vi "map other module channels.vi"(7 "instance id":string, 9 "channels":refnum<class "TBM channel.lvclass">[](array[class]), 10 "engine configuration in":refnum<class "engine configuration.lvclass">, 11 "TEC configuration in":refnum<class "TEC configuration.lvclass">) -> (0 "error out":errorcluster, 2 "engine configuration out":refnum<class "engine configuration.lvclass">, 3 "TEC configuration out":refnum<class "TEC configuration.lvclass">)   [LabVIEW 2013, in "TEC editor node.lvclass"]
uses:
  TEC editor node.lvclass
  <vilib>/NI/Module Execution Interface/Engine Configuration/engine configuration.lvclass
  configuration/TEC configuration.lvclass
  <vilib>/NI/Tag Bus Module Framework/channel/TBM channel.lvclass
  <vilib>/NI/Tag Bus Module Framework/channel/channel classification.ctl
  <vilib>/NI/Tag Bus Module Framework/channel/TBM channel.lvclass/TBM channel.ctl
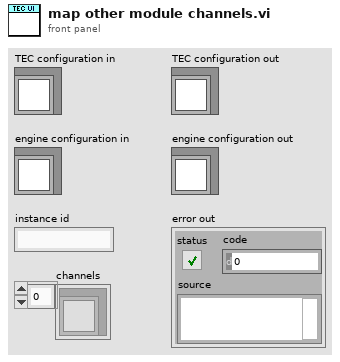
[diagram p1: front panel]
types:
  T1 = typedef "TBM channel.lvclass/channel classification.ctl" = enum16{"input data", "output data", "processing parameter", "processing result"}
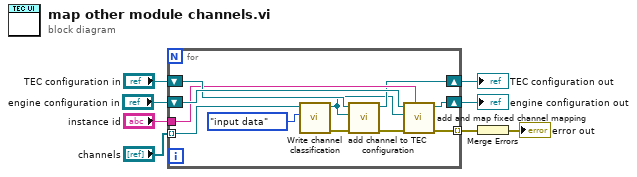
[diagram p0: block diagram]
diagram:
  n1 = for {
    tunnel: "channels" -> [w15] mode=indexing
    shift-right: [w16] -> w6
    shift-left: "TEC configuration in" -> [w18]
    tunnel: "instance id" -> [w17]
    tunnel: [w11] -> w5 mode=indexing
    shift-right: [w10] -> w7
    shift-left: "engine configuration in" -> [w19]
    n2 = call <vilib>:"Write channel classification.vi"("channel classification"=channel_classification."input data", "channel in"=w15) -> ("error out"=w12:errorcluster, "channel out"=w14:refnum<class "TBM channel.lvclass">)  [unwired: 8 in]
    n3 = call "add channel to TEC configuration.vi"("error in"=w12, "channel"=w14, "TEC configuration in"=w18) -> ("error out"=w13:errorcluster, "TEC configuration out"=w16:refnum<class "TEC configuration.lvclass">)  [unwired: 7 in]
    n4 = call <vilib>:"add and map fixed channel mapping.vi"("module instance"=w17, "error in"=w13, "fixed channel"=w14, "engine configuration in"=w19) -> ("error out"=w11:errorcluster, "engine configuration out"=w10:refnum<class "engine configuration.lvclass">)  [unwired: 6 in]
  }
  "engine configuration out" <- w7
  "TEC configuration out" <- w6
  n5 = Merge Errors(w5) -> (→"error out":errorcluster)
